vi "GetProperties.vi"(8 "error in":errorcluster, 11 "FPWindow in":refnum<class "FPWindow.lvclass">) -> (0 "error out":errorcluster, 3 "FPWindow out":refnum<class "FPWindow.lvclass">)   [LabVIEW 2014, in "Raspberry Pi Compatible Compiler for LabVIEW.lvlib" / "FPWindow.lvclass"]
uses:
  FPWindow.lvclass
  FPWindow.lvclass/FPWindow.ctl
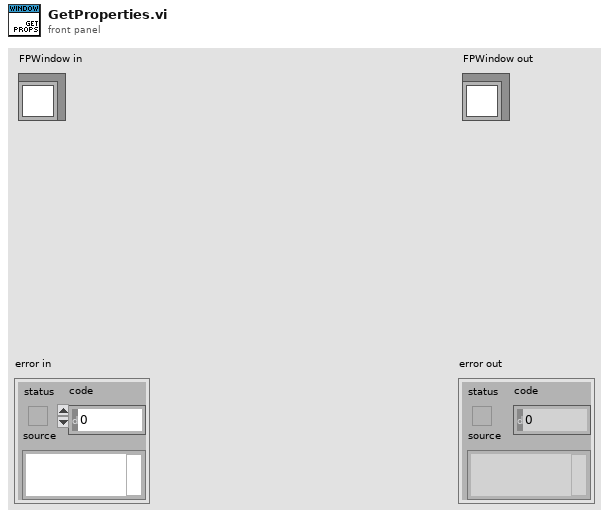
[diagram p1: front panel]
types:
  T1 = enum32{"Invalid", "Default", "Floating", "Floating/Auto-Hide", "Modal"}
  T2 = typedef "LVPointTypeDef.ctl" = cluster{"Horizontal":i16, "Vertical":i16}
  T3 = typedef "LVRectTypeDef.ctl" = cluster{"Left":i16, "Top":i16, "Right":i16, "Bottom":i16}
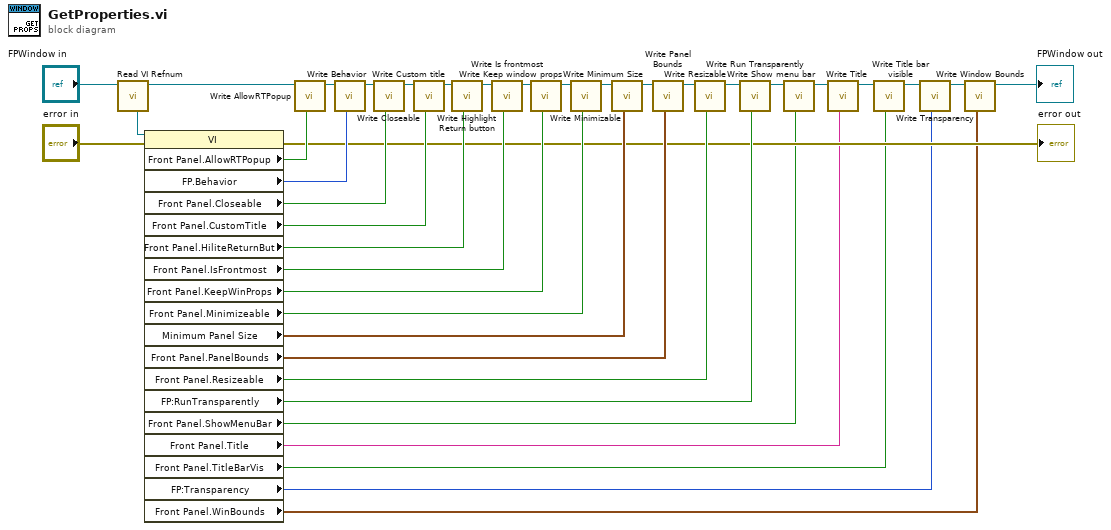
[diagram p0: block diagram]
diagram:
  n1 = call "Read VI Refnum.vi"("FPWindow in"="FPWindow in") -> ("FPWindow out"=w35:refnum<class "FPWindow.lvclass">, "VI Refnum"=w38:refnum<vi>)  [unwired: 7 in]
  n2 = property class="VI"(reference=w38, error in="error in") -> (error out=→"error out":errorcluster, "Front Panel.AllowRTPopup"=w36:bool, "FP.Behavior"=w33:T1, "Front Panel.Closeable"=w31:bool, "Front Panel.CustomTitle"=w29:bool, "Front Panel.HiliteReturnBut"=w27:bool, "Front Panel.IsFrontmost"=w25:bool, "Front Panel.KeepWinProps"=w24:bool, "Front Panel.Minimizeable"=w21:bool, "Minimum Panel Size"=w19:T2, "Front Panel.PanelBounds"=w17:T3, "Front Panel.Resizeable"=w15:bool, "FP:RunTransparently"=w13:bool, "Front Panel.ShowMenuBar"=w8:bool, "Front Panel.Title"=w7:string, "Front Panel.TitleBarVis"=w4:bool, "FP:Transparency"=w3:u8, "Front Panel.WinBounds"=w1:T3)  [unwired: 1 out]
  n3 = call "Write AllowRTPopup.vi"("AllowRTPopup"=w36, "FPWindow in"=w35) -> ("FPWindow out"=w34:refnum<class "FPWindow.lvclass">)  [unwired: 7 in]
  n4 = call "Write Behavior.vi"("Behavior"=w33, "FPWindow in"=w34) -> ("FPWindow out"=w32:refnum<class "FPWindow.lvclass">)  [unwired: 7 in]
  n5 = call "Write Closeable.vi"("Closeable"=w31, "FPWindow in"=w32) -> ("FPWindow out"=w30:refnum<class "FPWindow.lvclass">)  [unwired: 7 in]
  n6 = call "Write Custom title.vi"("Custom title"=w29, "FPWindow in"=w30) -> ("FPWindow out"=w28:refnum<class "FPWindow.lvclass">)  [unwired: 7 in]
  n7 = call "Write Highlight Return button.vi"("Highlight Return button"=w27, "FPWindow in"=w28) -> ("FPWindow out"=w26:refnum<class "FPWindow.lvclass">)  [unwired: 7 in]
  n8 = call "Write Is frontmost.vi"("Is frontmost"=w25, "FPWindow in"=w26) -> ("FPWindow out"=w23:refnum<class "FPWindow.lvclass">)  [unwired: 7 in]
  n9 = call "Write Keep window props.vi"("Keep window props"=w24, "FPWindow in"=w23) -> ("FPWindow out"=w22:refnum<class "FPWindow.lvclass">)  [unwired: 7 in]
  n10 = call "Write Minimizable.vi"("Minimizable"=w21, "FPWindow in"=w22) -> ("FPWindow out"=w20:refnum<class "FPWindow.lvclass">)  [unwired: 7 in]
  n11 = call "Write Minimum Size.vi"("Minimum Size"=w19, "FPWindow in"=w20) -> ("FPWindow out"=w18:refnum<class "FPWindow.lvclass">)  [unwired: 7 in]
  n12 = call "Write Panel Bounds.vi"("Panel Bounds"=w17, "FPWindow in"=w18) -> ("FPWindow out"=w16:refnum<class "FPWindow.lvclass">)  [unwired: 7 in]
  n13 = call "Write Resizable.vi"("Resizable"=w15, "FPWindow in"=w16) -> ("FPWindow out"=w14:refnum<class "FPWindow.lvclass">)  [unwired: 7 in]
  n14 = call "Write Run Transparently.vi"("Run Transparently"=w13, "FPWindow in"=w14) -> ("FPWindow out"=w12:refnum<class "FPWindow.lvclass">)  [unwired: 7 in]
  n15 = call "Write Show menu bar.vi"("Show menu bar"=w8, "FPWindow in"=w12) -> ("FPWindow out"=w6:refnum<class "FPWindow.lvclass">)  [unwired: 7 in]
  n16 = call "Write Title.vi"("Title"=w7, "FPWindow in"=w6) -> ("FPWindow out"=w5:refnum<class "FPWindow.lvclass">)  [unwired: 7 in]
  n17 = call "Write Title bar visible.vi"("Title bar visible"=w4, "FPWindow in"=w5) -> ("FPWindow out"=w2:refnum<class "FPWindow.lvclass">)  [unwired: 7 in]
  n18 = call "Write Transparency.vi"("Transparency"=w3, "FPWindow in"=w2) -> ("FPWindow out"=w11:refnum<class "FPWindow.lvclass">)  [unwired: 7 in]
  n19 = call "Write Window Bounds.vi"("Panel Bounds"=w1, "FPWindow in"=w11) -> ("FPWindow out"=→"FPWindow out":refnum<class "FPWindow.lvclass">)  [unwired: 7 in]
